vi "Check Is Test Case.vi"(11 "Path":path) -> (3 "Is Test Case?":bool)   [LabVIEW 2020, in "LUnit Test Suite.lvclass"]
uses:
  LUnit Test Suite.lvclass
  LUnit Test Case/LUnit Test Case.lvclass
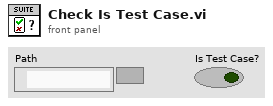
[diagram p1: front panel]
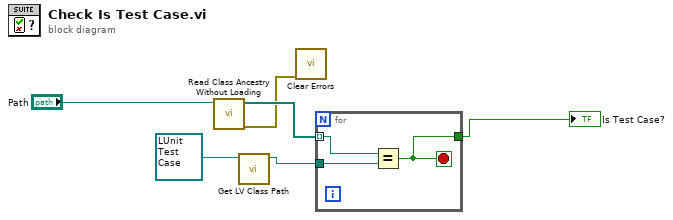
[diagram p0: block diagram]
diagram:
  n1 = call <vilib>:"Read Class Ancestry Without Loading.vi"("LabVIEW Class Path"="Path") -> ("error out"=w1:errorcluster, "Class Ancestry"=w3:path[])  [unwired: 9 in]
  n2 = call <vilib>:"Get LV Class Path.vi"("object"=refnum<class "LUnit Test Case.lvclass"> refnum ("LUnit Test Case V2.lvclass")) -> ("class path"=w6:path)  [unwired: 9 in, 1 out]
  n3 = call <vilib>:"Clear Errors.vi"("error in (no error)"=w1) -> ()  [unwired: 5 in, 2 out]
  n4 = for {
    tunnel: w3 -> [w8] mode=indexing
    tunnel: w6 -> [w9]
    tunnel: [w7] -> w4
    stop <- w7 stop-if-true
    n5 = Equal?(x=w8, y=w9) -> (x = y?=w7:bool)
  }
  "Is Test Case?" <- w4
